vi "Convert to Celsius.vi"(10 "Units in":T1, 11 "Value in":dbl) -> (2 "Units out":T1, 3 "Value out":dbl)   [LabVIEW 2019, in "2727.lvlib" / "2727.lvclass"]
uses:
  Library/2727.lvclass
  builds/Instruments/PRM.lvlibp/Custom Controls/Units.ctl
  builds/Instruments/PRM.lvlibp/Library/PRM.lvclass
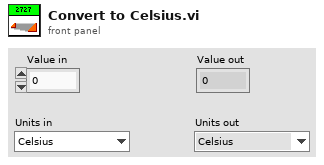
[diagram p1: front panel]
types:
  T1 = typedef "PRM.lvlibp/PRM.lvclass/Units.ctl" = enum16{"Celsius", "Fahrenheit", "Kelvin", "Ohms"}
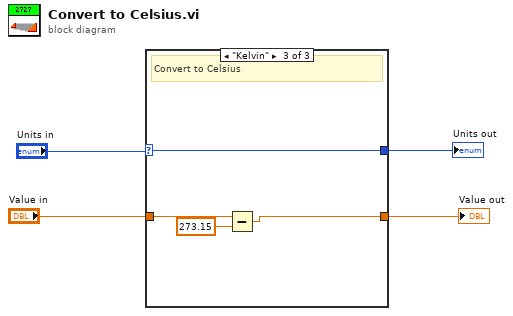
[diagram p0: block diagram]
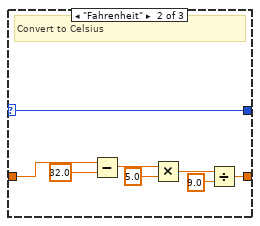
[diagram p3: hidden frame]
diagram:
  n1 = case shown="\"Kelvin\"" "Units in" {
    selector: "Units in" -> [w5 w7 w15]
    tunnel: "Value in" -> [w6 w14 w18]
    tunnel: [w6 w8 w16] -> w2
    tunnel: [w5 w7 w15] -> w1
    frame "Celsius", "Ohms" {
      # "Ohmic Setpoint or Already in Celsius"
    }
    frame "Fahrenheit" {
      # "Convert to Celsius"
      n2 = Subtract(x=w14, y=32.0) -> (x-y=w12:dbl)
      n3 = Multiply(x=w12, y=5.0 ("x")) -> (x*y=w9:dbl)
      n4 = Divide(x=w9, y=9.0) -> (x/y=w8:dbl)
    }
    frame "Kelvin" {
      # "Convert to Celsius"
      n5 = Subtract(x=w18, y=273.15) -> (x-y=w16:dbl)
    }
  }
  "Value out" <- w2
  "Units out" <- w1
